vi "Auto Turn Precise.vi"(7 "Target Distance":dbl=90.0 format="%#_13g", 8 "Error In":errorcluster, 11 "Refnum's In":T1) -> (0 "Error Out":errorcluster, 3 "Refnum's Out":T1)   [LabVIEW 2016]
uses:
  <vilib>/Rock Robotics/WPI/Utilities/WPI_GetSetVariantRefNum.vi
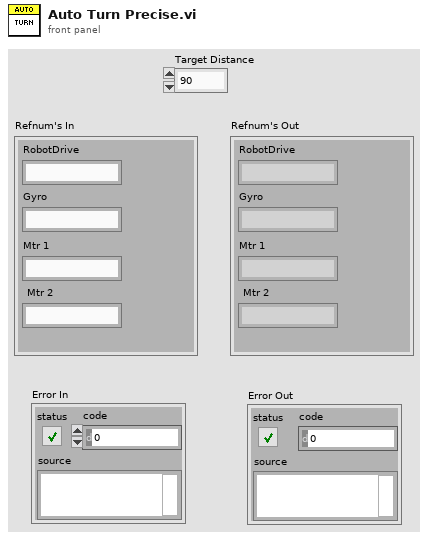
[diagram p1: front panel]
types:
  T1 = cluster{"RobotDrive":string, "Gyro":string, "Mtr 1":string, "Mtr 2":string}
  T2 = typedef "WPI_GyroDevRef.ctl" = cluster{"DevStatus":errorcluster, "Analog Channel":T3, "Offset":dbl, "Gain (VoltsPerDegree/Second)":dbl, "Gyro Type":enum16{"Analog", "XRS450"}, "Handle":i32, "SPI Bus":T4, "Device Found":bool, "Sample Rate":dbl, "Calibrate On Open":bool}
  T3 = typedef "FPGA_AIChannel.ctl" = enum8{"AI 0", "AI 1", "AI 2", "AI 3", "AI MXP 0", "AI MXP 1", "AI MXP 2", "AI MXP 3", "Invalid"}
  T4 = typedef "spi_bus.ctl" = enum16{"SPI On-Board, CS0", "SPI On-Board, CS1", "SPI On-Board, CS2", "SPI On-Board, CS3", "SPI MXP", "Invalid"}
  T5 = typedef "WPI_RobotDriveDevRef.ctl" = cluster{"DevStatus":errorcluster, "Motors[]":T6[], "Square Inputs":bool, "Max Output":dbl}
  T6 = typedef "WPI_MotorControlDeviceRef.ctl" = cluster{"DeviceStatus":errorcluster, "Type":T7, "PWM":cluster{"PWM Channel":T8, "DeadBand":T9}, "CAN":cluster{"Device Number":u8, "SetOutput VI Ref":variant, "GetOutput VI Ref":variant, "Enable VI Ref":variant, "Disable VI Ref":variant, "Data":variant}, "Invert":bool}
  T7 = typedef "WPI_MotorControlType.ctl" = enum16{"PWM", "CAN"}
  T8 = typedef "FPGA_DIOPWMChannel.ctl" = enum8{"PWM 0", "PWM 1", "PWM 2", "PWM 3", "PWM 4", "PWM 5", "PWM 6", "PWM 7", "PWM 8", "PWM 9", "PWM MXP 0", "PWM MXP 1", "PWM MXP 2", "PWM MXP 3", "PWM MXP 4", "PWM MXP 5", "PWM MXP 6", "PWM MXP 7", "PWM MXP 8", "PWM MXP 9", "Invalid"}
  T9 = typedef "WPI_PWMDeadband.ctl" = cluster{"Name":string, "maxPositivePwm":i32, "minPositivePwm":i32, "centerPwm":i32, "maxNegativePwm":i32, "minNegativePwm":i32, "angularRange":u16}
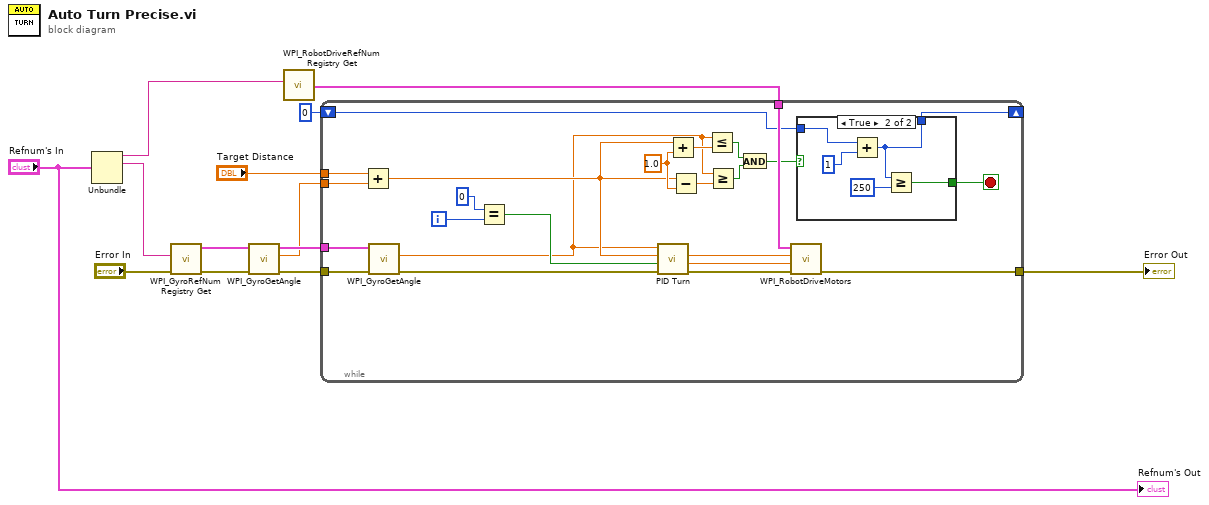
[diagram p0: block diagram]
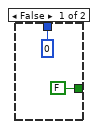
[diagram p2: hidden frame]
diagram:
  n1 = Unbundle("Refnum's In") -> ("RobotDrive"=w8:string, "Gyro"=w7:string)  [unwired: 2 out]
  n2 = call <vilib>:"WPI_GyroRefNum Registry Get.vi"("error in (no error)"="Error In", "refnum name"=w7) -> ("error out"=w10:errorcluster, "GyroDevRef"=w11:T2)  [unwired: 8 in]
  n3 = call <vilib>:"WPI_GyroGetAngle.vi"("error in"=w10, "GyroDevRef"=w11) -> ("error out"=w3:errorcluster, "Angle"=w2:dbl, "GyroDevRef"=w4:T2)  [unwired: 5 in, 2 out]
  n4 = call <vilib>:"WPI_RobotDriveRefNum Registry Get.vi"("refnum name"=w8) -> ("RobotDriveDevRef"=w13:T5)  [unwired: 9 in, 1 out]
  n5 = while {
    tunnel: w13 -> [w35]
    tunnel: w4 -> [w34]
    tunnel: w3 -> [w33]
    shift-right: [w26] -> _
    shift-left: 0 -> [w25]
    tunnel: "Target Distance" -> [w19]
    tunnel: [w20] -> w5
    tunnel: w2 -> [w18]
    i -> [w37]
    stop <- w14 stop-if-true
    w32 = 1.0 ("y")
    n6 = Add(x=w19, y=w18) -> (x+y=w17:dbl)
    n7 = call <vilib>:"WPI_GyroGetAngle.vi"("error in"=w33, "GyroDevRef"=w34) -> ("error out"=w16:errorcluster, "Angle"=w15:dbl)  [unwired: 5 in, 3 out]
    n8 = Equal?(x=0, y=w37) -> (x = y?=w24:bool)
    n9 = call "PID Turn.vi"("Error In"=w16, "Reinitialize"=w24, "Target Angle"=w17, "Gyro Angle"=w15) -> ("Error Out"=w23:errorcluster, "Right Power"=w22:dbl, "Left Power"=w21:dbl)  [unwired: 5 in]
    n10 = Add(x=w17, y=w32) -> (x+y=w31:dbl)
    n11 = Subtract(x=w17, y=w32) -> (x-y=w30:dbl)
    n12 = Less Or Equal?(x=w15, y=w31) -> (x <= y?=w29:bool)
    n13 = Greater Or Equal?(x=w15, y=w30) -> (x >= y?=w28:bool)
    n14 = And(x=w29, y=w28) -> (x .and. y?=w27:bool)
    n15 = call <vilib>:"WPI_RobotDriveMotors.vi"("error in (no error)"=w23, "RightSpeed"=w22, "LeftSpeed"=w21, "RobotDriveDevRef"=w35) -> ("error out"=w20:errorcluster)  [unwired: 5 in, 2 out]
    n16 = case shown="True" w27 {
      tunnel: w25 -> [_ w43]
      tunnel: [0 w42] -> w26
      tunnel: [FALSE w40] -> w14
      frame False {
      }
      frame True {
        n17 = Add(x=w43, y=1) -> (x+y=w42:i32)
        n18 = Greater Or Equal?(x=w42, y=250) -> (x >= y?=w40:bool)
      }
    }
  }
  "Error Out" <- w5
  "Refnum's Out" <- "Refnum's In"
